vi "remote.Read Dev.ProductCategory.vi"(8 "error in (no error)":errorcluster, 11 "SLSC Remote in":refnum<class "SLSC Interface.lvclass">) -> (0 "error out":errorcluster, 2 "Dev.ProductCategory":i32(ring) items=["Unknown", "SLSC Chassis", "SLSC Module"], 3 "SLSC Remote out":refnum<class "SLSC Interface.lvclass">)   [LabVIEW 2016, in "SLSC Interfaces.lvlib" / "SLSC Interface.lvclass"]
uses:
  SLSC Interface Class/SLSC Interface.lvclass
  <vilib>/NI/JSON Support for LabVIEW/JSON Data Classes/JSON Helper/JSON Helper.lvclass
  <vilib>/NI/JSON Support for LabVIEW/JSON Data Classes/JSON Helper/To More Specific Type (Numeric).vi
  <vilib>/NI/JSON Support for LabVIEW/JSON Data Classes/JSON Basic Type/JSON Literal.lvclass
  <vilib>/NI/JSON Support for LabVIEW/JSON Data Classes/JSON Numeric/Read value (Numeric).vi
  <vilib>/NI/JSON Support for LabVIEW/JSON Data Classes/JSON Numeric/JSON Numeric.lvclass
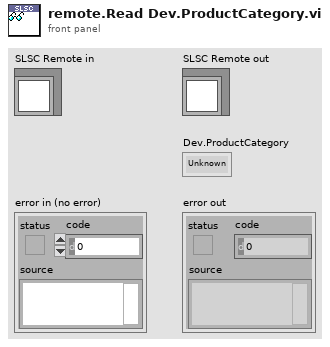
[diagram p1: front panel]
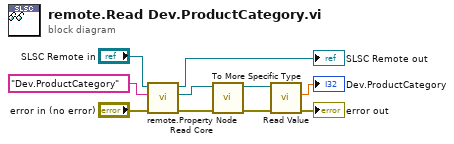
[diagram p0: block diagram]
diagram:
  n1 = call "remote.Property Node Read Core.vi"("error in (no error)"="error in (no error)", "property"="Dev.ProductCategory", "SLSC Remote in"="SLSC Remote in") -> ("error out"=w6:errorcluster, "value"=w5:refnum<class "JSON Null.lvclass">, "SLSC Remote out"=→"SLSC Remote out":refnum<class "SLSC Interface.lvclass">)  [unwired: 6 in]
  n2 = call-poly <vilib>:"To More Specific Type.vi"("error in (no error)"=w6, "JSON Datatype in"=w5) -> ("error out"=w1:errorcluster, "JSON Numeric out"=w4:refnum<class "JSON Numeric.lvclass">)  [unwired: 8 in]
  n3 = call-poly <vilib>:"Read Value.vi"("error in (no error)"=w1, "JSON Numeric in"=w4) -> ("error out"=→"error out":errorcluster, "value"=→"Dev.ProductCategory":dbl)  [unwired: 8 in]
